vi "Byte Mask.vi"(9 "Byte Mask":u8 format="%08b", 11 "Data":u32 format="%08x") -> (1 "Masked Data":u32 format="%08x")   [LabVIEW 2011]
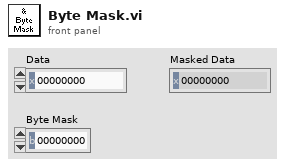
[diagram p1: front panel]
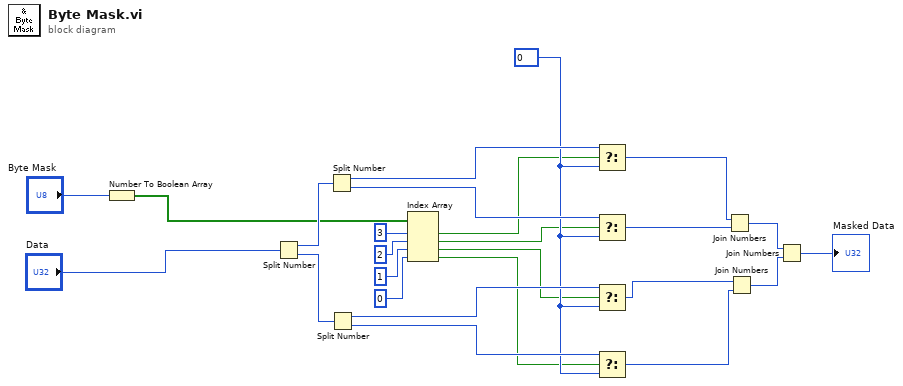
[diagram p0: block diagram]
diagram:
  w9 = i8 0 ("f")
  n1 = Number To Boolean Array(number="Byte Mask") -> (Boolean array=w14:bool[])
  n2 = Split Number(x="Data") -> (hi(x)=w24:u16, lo(x)=w23:u16)
  n3 = Split Number(x=w24) -> (hi(x)=w13:u8, lo(x)=w12:u8)
  n4 = Split Number(x=w23) -> (hi(x)=w11:u8, lo(x)=w10:u8)
  n5 = Index Array(array=w14, index #1=3 ("index"), index #2=2 ("index"), index #3=1 ("index"), index #4=0 ("index")) -> (element #1=w4:bool, element #2=w3:bool, element #3=w2:bool, element #4=w1:bool)
  n6 = Select(t=w13, s=w4, f=w9) -> (s? t:f=w16:u8)
  n7 = Select(t=w12, s=w3, f=w9) -> (s? t:f=w17:u8)
  n8 = Select(t=w11, s=w2, f=w9) -> (s? t:f=w18:u8)
  n9 = Select(t=w10, s=w1, f=w9) -> (s? t:f=w19:u8)
  n10 = Join Numbers(hi=w16, lo=w17) -> ((hi.lo)=w21:u16)
  n11 = Join Numbers(hi=w18, lo=w19) -> ((hi.lo)=w20:u16)
  n12 = Join Numbers(hi=w21, lo=w20) -> ((hi.lo)=→"Masked Data":u32)
